vi "writePIDSetting.vi"(8 "Error In":errorcluster, 9 "Ch3 PID gains":T1={"proportional gain (Kc)"=0.5, "integral time (Ti, min)"=0.0003, "derivative time (Td, min)"=1e-05} {"derivative time (Td, min)" format="%.5f"; "integral time (Ti, min)" format="%.5f"; "proportional gain (Kc)" format="%.3f"}, 10 "Ch2 PID gains":T1={"proportional gain (Kc)"=0.5, "integral time (Ti, min)"=0.0003, "derivative time (Td, min)"=1e-05} {"derivative time (Td, min)" format="%.5f"; "integral time (Ti, min)" format="%.5f"; "proportional gain (Kc)" format="%.3f"}, 11 "Ch1 PID gains":T1={"proportional gain (Kc)"=0.5, "integral time (Ti, min)"=0.0003, "derivative time (Td, min)"=1e-05} {"derivative time (Td, min)" format="%.5f"; "integral time (Ti, min)" format="%.5f"; "proportional gain (Kc)" format="%.3f"}) -> (0 "Error Out":errorcluster)   [LabVIEW 2020]
uses:
  <vilib>/Utility/config.llb/Write Key (Double).vi
  <vilib>/Utility/config.llb/NI_LVConfig.lvlib
panel:
  out "Setting file path":path
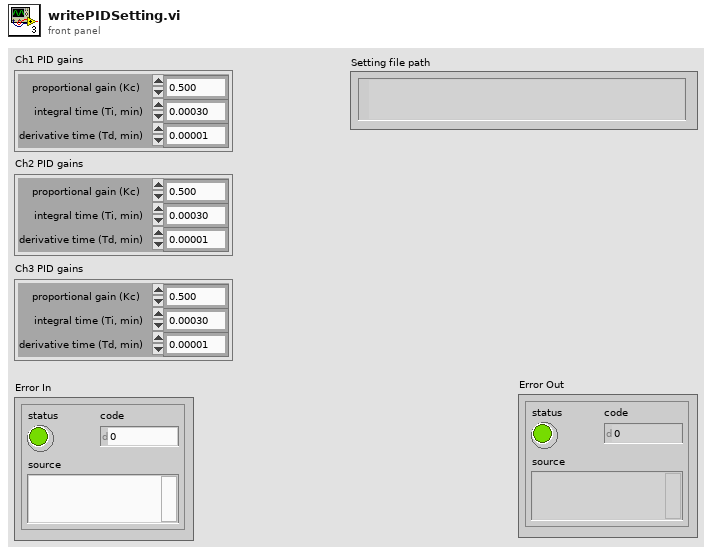
[diagram p1: front panel]
types:
  T1 = cluster{"proportional gain (Kc)":dbl, "integral time (Ti, min)":dbl, "derivative time (Td, min)":dbl}
  T2 = cluster{"proportional gain (Kc)":dbl, "integral time (Ti, min)":dbl, "derivative time (Td, min)":dbl}[]
  T3 = typedef "NI_LVConfig.lvlib/Config Data RefNum.ctl" = refnum<k1>
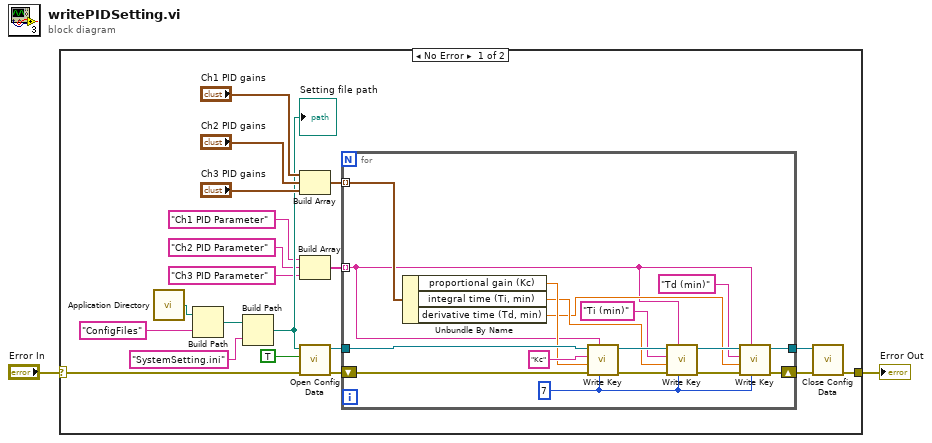
[diagram p0: block diagram]
diagram:
  n1 = case shown="No Error" "Error In" {
    selector: "Error In" -> [w14 w40]
    tunnel: [w3 w40] -> w1
    frame No Error {
      n2 = call <vilib>:"Application Directory.vi"() -> ("Application Directory"=w22:path)
      n3 = Build Path(base path=w22, name or relative path="ConfigFiles") -> (appended path=w20:path)
      n4 = Build Path(base path=w20, name or relative path="SystemSetting.ini") -> (appended path=w13:path)
      "Setting file path" <- w13
      n5 = Build Array("Ch1 PID gains", "Ch2 PID gains", "Ch3 PID gains") -> (w6:T2)
      n6 = Build Array("Ch1 PID Parameter", "Ch2 PID Parameter", "Ch3 PID Parameter") -> (w7:string[])
      n7 = call <vilib>:"Open Config Data.vi"("error in (no error)"=w14, "create file if necessary (T)"=TRUE, "configuration file path"=w13) -> ("error out"=w11:errorcluster, "refnum"=w12:T3)  [unwired: 6 in, 1 out]
      n8 = for {
        tunnel: w12 -> [w39]
        shift-right: [w24] -> w4
        shift-left: w11 -> [w38]
        tunnel: w7 -> [w25] mode=indexing
        tunnel: w6 -> [w34] mode=indexing
        tunnel: [w23] -> w5
        w26 = i16 7 ("precision (6)")
        n9 = Unbundle By Name(w34) -> ("proportional gain (Kc)"=w29:dbl, "integral time (Ti, min)"=w28:dbl, "derivative time (Td, min)"=w27:dbl)
        n10 = call-poly <vilib>:"Write Key.vi"("precision (6)"=w26, "section"=w25, "error in (no error)"=w38, "value"=w29, "key"="Kc", "refnum"=w39) -> ("error out"=w35:errorcluster, "refnum out"=w36:T3)  [unwired: 3 in, 1 out]
        n11 = call-poly <vilib>:"Write Key.vi"("precision (6)"=w26, "section"=w25, "error in (no error)"=w35, "value"=w28, "key"="Ti (min)", "refnum"=w36) -> ("error out"=w31:errorcluster, "refnum out"=w32:T3)  [unwired: 3 in, 1 out]
        n12 = call-poly <vilib>:"Write Key.vi"("precision (6)"=w26, "section"=w25, "error in (no error)"=w31, "value"=w27, "key"="Td (min)", "refnum"=w32) -> ("error out"=w24:errorcluster, "refnum out"=w23:T3)  [unwired: 3 in, 1 out]
      }
      n13 = call <vilib>:"Close Config Data.vi"("error in (no error)"=w4, "refnum"=w5) -> ("error out"=w3:errorcluster)  [unwired: 8 in, 1 out]
    }
    frame Error {
    }
  }
  "Error Out" <- w1
